vi "IM-RT_gui2.vi"() -> ()   [LabVIEW 2017]
uses:
  <userlib>/_OpalApi/Code/Code/Clients/labview/distribution/api/OpalApi.lvlib
panel:
  out "Rotor Current (Amps)":dbl[](graph)
  out "Stator Current (Amps)":dbl[](graph)
  out "Inertia":dbl
  out "Lm (H)":dbl
  out "Number of Poles":dbl
  out "Lr (H)":dbl
  out "Rr (Ohm)":dbl
  out "Ls (H)":dbl
  out "Rs (Ohm)":dbl
  out "Vc":dbl[](graph)
  out "Vb":dbl[](graph)
  in  "Grid Voltage Amp":dbl(knob) scale=0.0..400.0
  out "Torque output":dbl[](graph)
  out "Running":bool
  in  "Load Torque":dbl[](array[slide]) scale=0.0..150.0
  out "Va":dbl[](graph)
  out "Gauge":dbl(knob) scale=0.0..3600.0 scale format="%#_5g"
  # "Motor Parameters"
  # "Speed"
  # "Grid Input - Phase A"
  # "Grid Input - Phase B"
  # "Grid Input - Phase C"
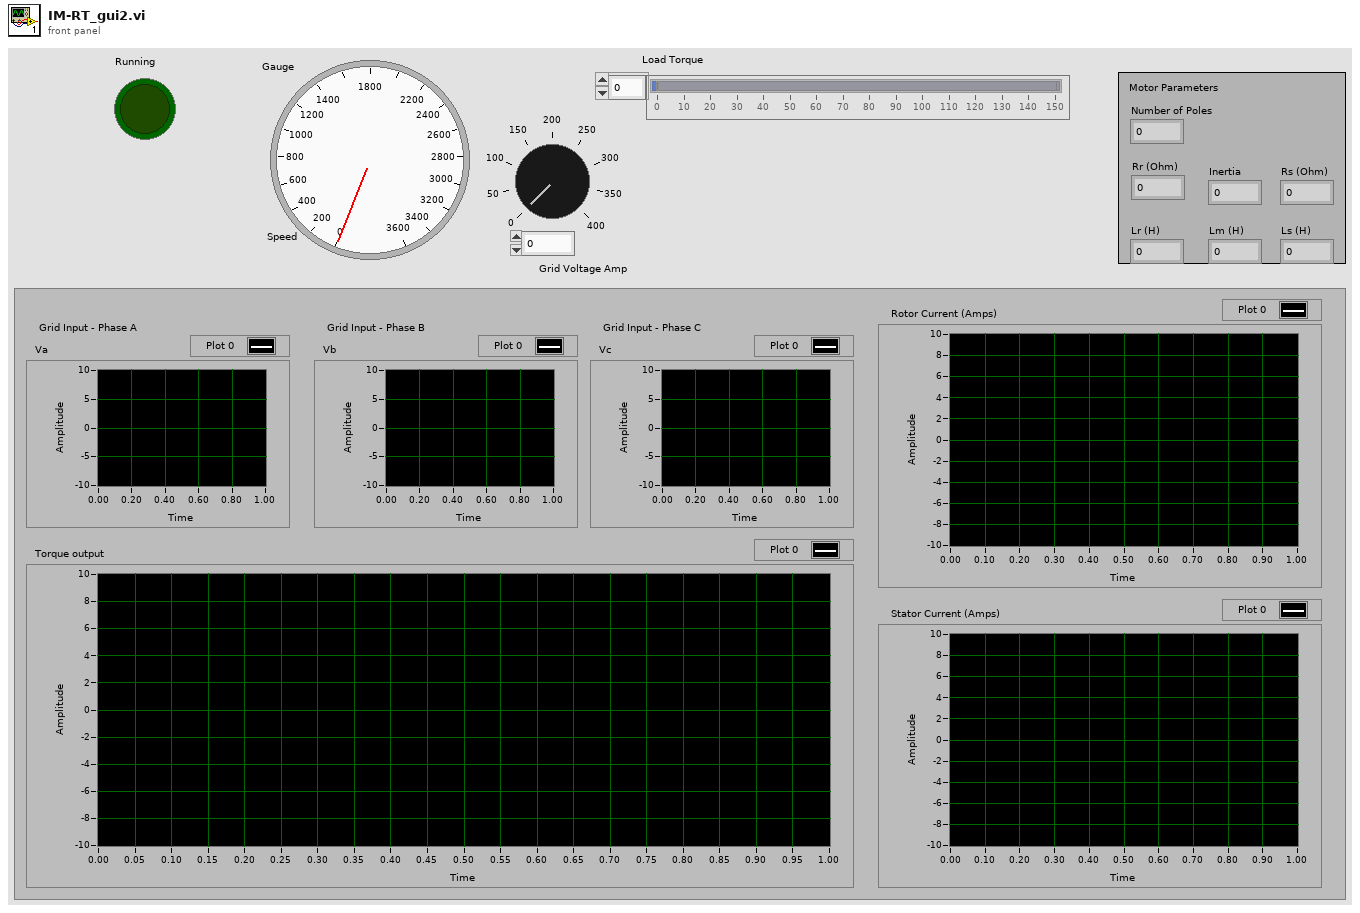
[diagram p1: front panel]
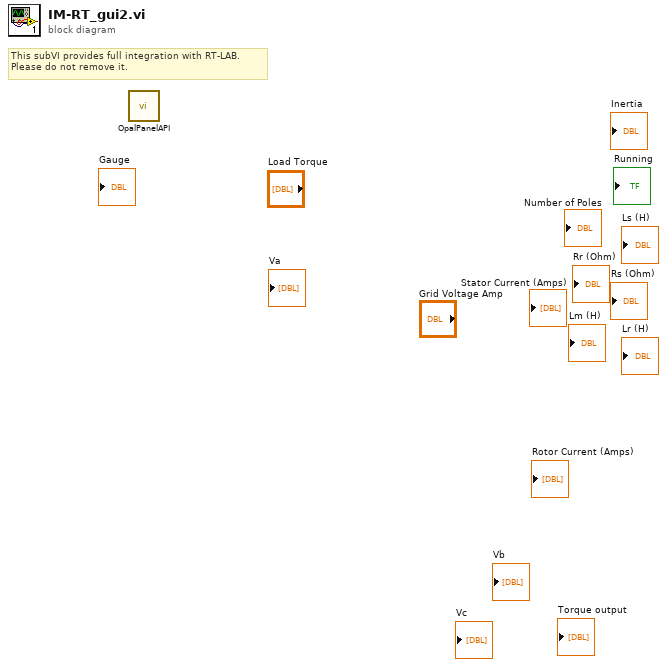
[diagram p0: block diagram]
diagram:
  # "This subVI provides full integration with RT-LAB.\nPlease do not remove it."
  n1 = call <userlib>:"OpalPanelAPI.vi"() -> ()  [unwired: 1 in]
